vi "Initialize Output DMA Refs.vi"(8 "error in (no error)":errorcluster, 10 "Settings.Compiled":T1 {"IncomingRegisters.Settings"."Register"."Data Type" format="%.0x"; "IncomingRegisters.Refs"."Refs"."Data Reference" format="%.0x"; "OutgoingRegisters.Settings"."Register"."Data Type" format="%.0x"; "OutgoingRegisters.Refs"."Refs"."Data Reference" format="%.0x"; "IncomingDMA.Settings"."DMA.Settings"."dt" format="%#_p"; "IncomingDMA.Settings"."DMA.Settings"."Update Rate" items=["1 Hz"=1, "2 Hz"=2, "5 Hz"=5, "10 Hz"=10]; "OutgoingDMA.Settings"."DMA.Settings"."dt" format="%#_p"; "OutgoingDMA.Settings"."DMA.Settings"."Update Rate" items=["1 Hz"=1, "2 Hz"=2, "5 Hz"=5, "10 Hz"=10]}, 11 "FPGA Ref":refnum<k20>) -> (0 "error out":errorcluster, 2 "DMA":T15[](array[typedef]), 3 "FPGA Ref":refnum<k20>)   [LabVIEW 2015, in "FPGA Addon Engine.lvlib"]
uses:
  FPGA Addon Engine.lvlib
  Types/DMA Output References.ctl
  <vilib>/NI VeriStand/Custom Device Waveform API/Single Waveform Read (DBL)/Single Waveform Read (DBL).lvclass
  Types/DMA Output Ref.ctl
  Shared/Compiled.Settings
  Shared/Compiled.RegisterSettings.ctl
  Shared/Scalar Type.ctl
  Shared/Register Information.ctl
  Shared/Data Type.ctl
  <vilib>/NI Veristand/Custom Device API/Block Data Reference.ctl
  <vilib>/NI Veristand/Custom Device API/Data Reference.ctl
  Shared/Compiled.DMASettings.ctl
  Shared/DMA Settings.ctl
  Shared/Delacing Scheme.ctl
  Shared/DMA Acquisition Mode.ctl
  <vilib>/NI Veristand/Custom Device API/Waveform Data Reference.ctl
  Shared/FPGA Settings.ctl
  <vilib>/NI Veristand/Custom Device API/Custom Device Target Type.ctl
  <vilib>/NI/LVFPGA Adv Session Resources/OpenByNameSubVI.vi
  <vilib>/NI Veristand/Custom Device Waveform API/Single Waveform Read (DBL)/NI VeriStand - Open Single Waveform Read Session (DBL).vi
  <vilib>/Utility/error.llb/Error Cluster From Error Code.vi
  <vilib>/rvi/interface/common/niFpgaWaitOnOcc.vi
  <vilib>/rvi/interface/common/dynamic/niFpgaEscapeDelimiterAndNull.vi
  <vilib>/rvi/interface/nirviMethod/nirviMethod.xnode
  <vilib>/NI/LVFPGA Adv Session Resources/OpenByName.xnode
  <vilib>/NI Veristand/Custom Device Waveform API/NI_VS Custom Device Waveform API.lvlib
  <vilib>/rvi/errors/niLvFpgaMergeErrorWithErrorCode.vi
  <vilib>/FPGAPlugInAG/Dynamic/niLvFpga_ConfigureFifo_Dynamic.vi
  <vilib>/FPGAPlugInAG/Dynamic/niLvFpga_StartFifo_Dynamic.vi
  <vilib>/NI/LVFPGA Adv Session Resources/LVFPGAAdvSessionResources.lvlib
  <vilib>/NI Veristand/Custom Device API/Custom Device API.lvlib
  Shared/FPGA Addon Shared.lvlib
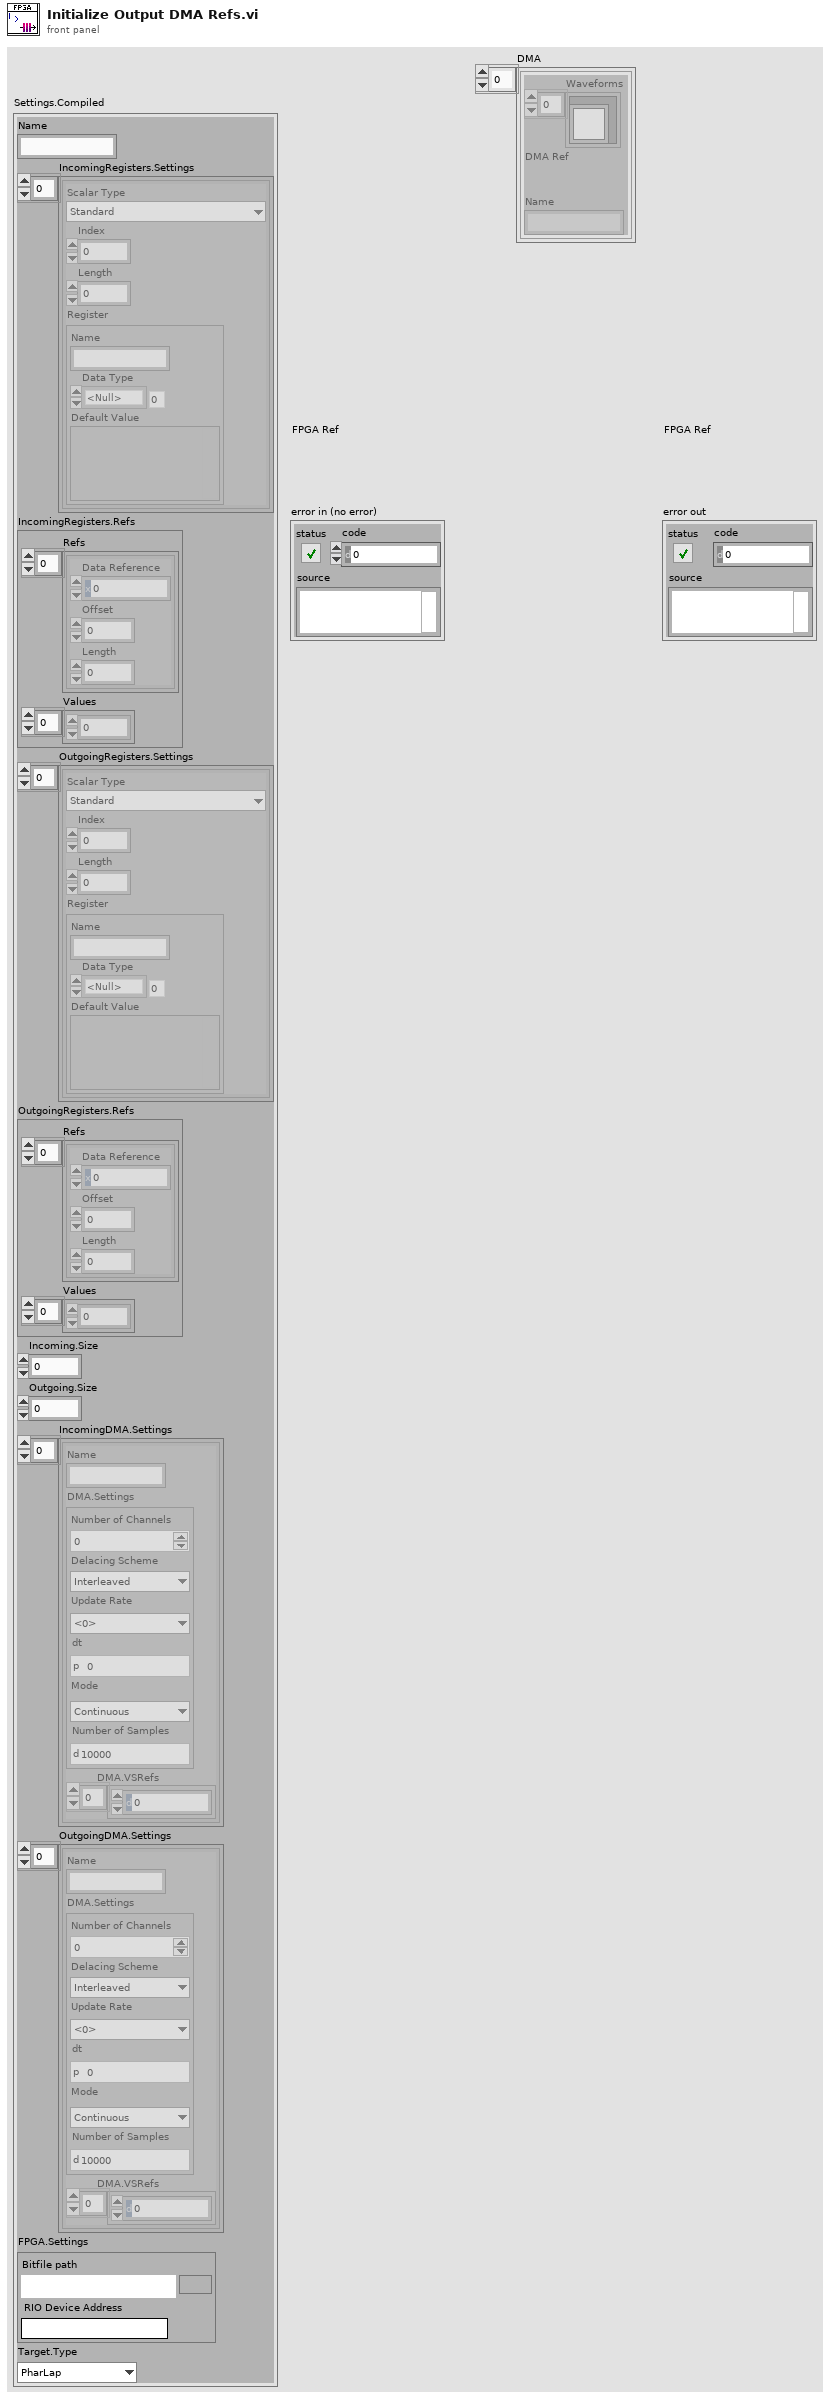
[diagram p1: front panel]
types:
  T1 = typedef "FPGA Addon Shared.lvlib/Compiled.Settings" = cluster{"Name":string, "IncomingRegisters.Settings":T2[], "IncomingRegisters.Refs":cluster{"Refs":T6[], "Values":dbl[]}, "OutgoingRegisters.Settings":T2[], "OutgoingRegisters.Refs":cluster{"Refs":T6[], "Values":dbl[]}, "Incoming.Size":i32, "Outgoing.Size":i32, "IncomingDMA.Settings":T8[], "OutgoingDMA.Settings":T8[], "FPGA.Settings":T13, "Target.Type":T14}
  T2 = typedef "FPGA Addon Shared.lvlib/Compiled.RegisterSettings.ctl" = cluster{"Scalar Type":T3, "Index":i32, "Length":i32, "Register":T4}
  T3 = typedef "FPGA Addon Shared.lvlib/Scalar Type.ctl" = enum16{"Standard", "Bitpacked"}
  T4 = typedef "FPGA Addon Shared.lvlib/Register Information.ctl" = cluster{"Name":string, "Data Type":T5, "Default Value":variant}
  T5 = typedef "FPGA Addon Shared.lvlib/Data Type.ctl" = enum8{"<Null>", "I8", "I16", "I32", "I64", "U8", "U16", "U32", "U64", "SGL", "Boolean", "Analog PWM In Settings", "Analog PWM In", "Digital PWM In Settings", "Digital PWM In", "Digital PWM Out"}
  T6 = typedef "Custom Device API.lvlib/Block Data Reference.ctl" = cluster{"Data Reference":T7, "Offset":u64, "Length":u64}
  T7 = typedef "Custom Device API.lvlib/Data Reference.ctl" = i32
  T8 = typedef "FPGA Addon Shared.lvlib/Compiled.DMASettings.ctl" = cluster{"Name":string, "DMA.Settings":T9, "DMA.VSRefs":T12[]}
  T9 = typedef "FPGA Addon Shared.lvlib/DMA Settings.ctl" = cluster{"Number of Channels":u8, "Delacing Scheme":T10, "Update Rate":u32, "dt":dbl, "Mode":T11, "Number of Samples":u32}
  T10 = typedef "FPGA Addon Shared.lvlib/Delacing Scheme.ctl" = enum8{"Interleaved"}
  T11 = typedef "FPGA Addon Shared.lvlib/DMA Acquisition Mode.ctl" = enum8{"Continuous", "Triggered Finite"}
  T12 = typedef "Custom Device API.lvlib/Waveform Data Reference.ctl" = i32
  T13 = typedef "FPGA Addon Shared.lvlib/FPGA Settings.ctl" = cluster{"Bitfile path":path, "RIO Device Address":string}
  T14 = typedef "Custom Device API.lvlib/Custom Device Target Type.ctl" = enum16{"PharLap", "VxWorks", "Windows", "Linux_32_ARM", "Linux_x64"}
  T15 = typedef "FPGA Addon Engine.lvlib/DMA Output References.ctl" = cluster{"Waveforms":refnum<class "Single Waveform Read (DBL).lvclass">[], "DMA Ref":T16, "Name":string}
  T16 = typedef "FPGA Addon Engine.lvlib/DMA Output Ref.ctl" = refnum<k20>
  T17 = cluster{"Name":string, "Depth":u32, "Write? (Deprecated:Use Implementation)":bool, "Physical Channel":u32, "Base Address":u32, "Data Width":u32, "Data Type":enum32{"Boolean", "I8", "I16", "I32", "I64", "U8", "U16", "U32", "U64", "FXP", "CustomControl", "SGL"}, "FXP Properties":variant, "Write Window Address":u32, "Implementation":enum16{"niFpgaTargetToHost", "niFpgaHostToTarget", "niFpgaPeerToPeerWriter", "niFpgaPeerToPeerReader", "niCoreTargetToHost", "niCoreHostToTarget"}, "Control Set":u32}[]
  T18 = cluster{"Name":string, "type":variant, "indicator?":bool}[]
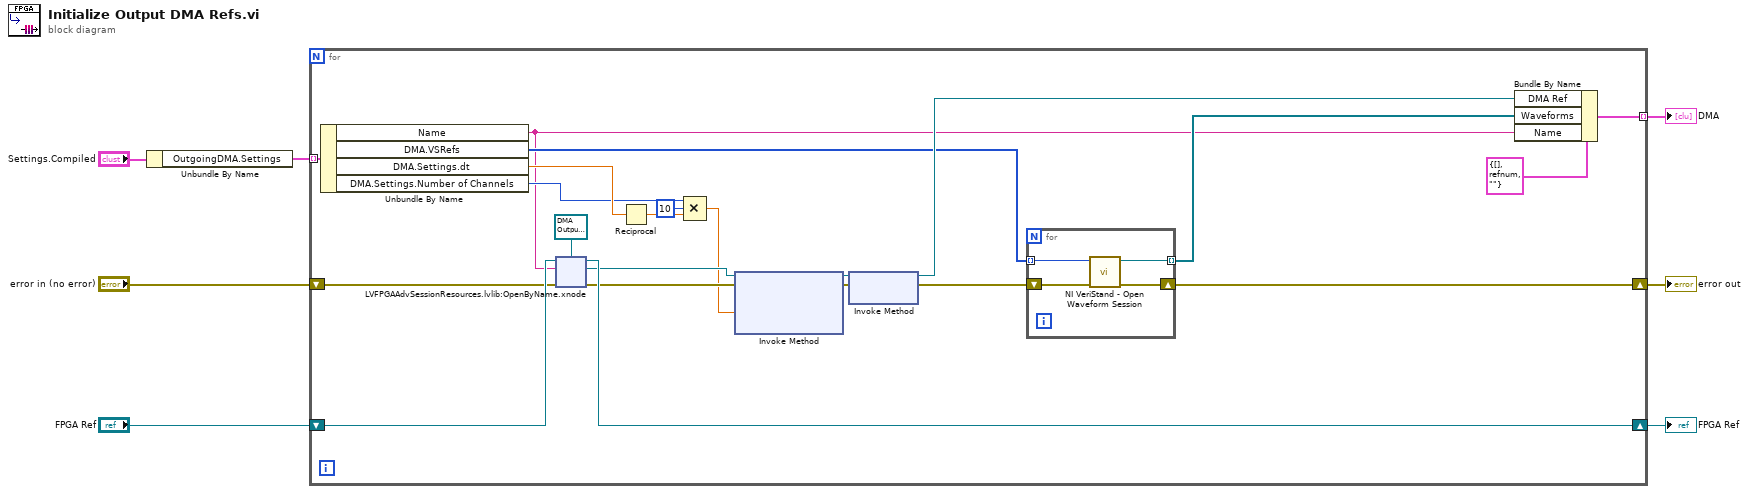
[diagram p0: block diagram]
diagram:
  n1 = Unbundle By Name("Settings.Compiled") -> ("OutgoingDMA.Settings"=w2:T8[])
  n2 = for {
    shift-right: [w8] -> w5
    shift-left: "error in (no error)" -> [w14]
    shift-right: [w27] -> w6
    shift-left: "FPGA Ref" -> [w28]
    tunnel: [w25] -> w4 mode=indexing
    tunnel: w2 -> [w16] mode=indexing
    n3 = Unbundle By Name(w16) -> ("Name"=w10:string, "DMA.VSRefs"=w15:T12[], "DMA.Settings.dt"=w13:dbl, "DMA.Settings.Number of Channels"=w12:u8)
    n4 = xnode "LVFPGAAdvSessionResources.lvlib:OpenByName.xnode"("FPGA VI Reference in"=w28, "Resource name in"=w10, "Single resource reference type in"=T16 refnum, "Error in"=w14) -> ("Single resource reference out"=w21:T16, "Error out"=w22:errorcluster, "FPGA VI Reference out"=w27:refnum<k20>)
    n5 = Reciprocal(x=w13) -> (1/x=w20:dbl)
    n6 = Compound Arithmetic op=MULTIPLY(w12, u8 10 ("value"), w20) -> (w17:dbl)
    n7 = xnode "Invoke Method"("FPGA VI Reference In"=w21, "error in"=w22, "Requested Depth"=w17) -> ("FPGA VI Reference Out"=w24:T16, "error out"=w23:errorcluster)  [unwired: 1 out]
    n8 = xnode "Invoke Method"("FPGA VI Reference In"=w24, "error in"=w23) -> ("FPGA VI Reference Out"=w18:T16, "error out"=w9:errorcluster)
    n9 = for {
      shift-right: [w33] -> w8
      shift-left: w9 -> [w31]
      tunnel: [w32] -> w11 mode=indexing
      tunnel: w15 -> [w30] mode=indexing
      n10 = call-poly <vilib>:"NI VeriStand - Open Waveform Session.vi"("error in (no error)"=w31, "DBL Waveform Data Reference"=w30) -> ("error out"=w33:errorcluster, "Single Waveform Read Session (DBL)"=w32:refnum<class "Single Waveform Read (DBL).lvclass">)  [unwired: 8 in]
    }
    n11 = Bundle By Name(cluster=T15 {"Waveforms"=[], "DMA Ref"=refnum, "Name"=""}, "DMA Ref"=w18, "Waveforms"=w11, "Name"=w10) -> (w25:T15)
  }
  "error out" <- w5
  "FPGA Ref" <- w6
  "DMA" <- w4
